vi "AFM_sync_fixed_lightsheet.vi"() -> ()   [LabVIEW 2017]
uses:
  <vilib>/DAQmx/write.llb/DAQmx Write (Analog DBL 1Chan 1Samp).vi
  <vilib>/DAQmx/write.llb/DAQmx Write (Analog 2D DBL NChan NSamp).vi
  <vilib>/DAQmx/create/channels.llb/DAQmx Create Channel (AO-Voltage-Basic).vi
  <vilib>/DAQmx/miscellaneous.llb/DAQmx Fill In Error Info.vi
  <vilib>/DAQmx/create/channels.llb/DAQmx Create Channel (CO-Pulse Generation-Frequency).vi
  <vilib>/DAQmx/configure/timing.llb/DAQmx Timing (Implicit).vi
  <vilib>/DAQmx/configure/trigger.llb/DAQmx Start Trigger (Digital Edge).vi
  <vilib>/DAQmx/configure/timing.llb/DAQmx Timing (Sample Clock).vi
  <resource>/objmgr/daqmx.rc
panel:
  in  "Unit Time":dbl=100.0 caption="ms" format="%#_13g"
  in  "ETL3 (V)  (4.76V allows light passing through unaltered.)":dbl(slide)=4.76 caption="ETL3 (dpt)" min=-12.029999732971191 max=16.450000762939453 step=0.009999999776482582 scale=0.0..10.0
  out "Focal Distance (um)":dbl
  out "Diopter":dbl
  in  "Blanking (0-10V)":dbl=10.0 min=0.0 max=10.0 step=0.1 format="%#_13g"
  in  "561 (0-10V)":dbl=2.0 min=0.0 max=10.0 step=0.1 format="%#_13g"
  in  "488 (0-10V)":dbl=2.0 min=0.0 max=10.0 step=0.1 format="%#_13g"
  out "Matched AFM frequency":dbl caption="frames/s"
  in  "OFF Time Unit":dbl=1.0 caption="(400 ms)" format="%#_13g"
  in  "ON Time Unit":dbl=3.0 caption="(600 ms)" format="%#_13g"
  # "(There is a hidden -1ms in Unit Time)"
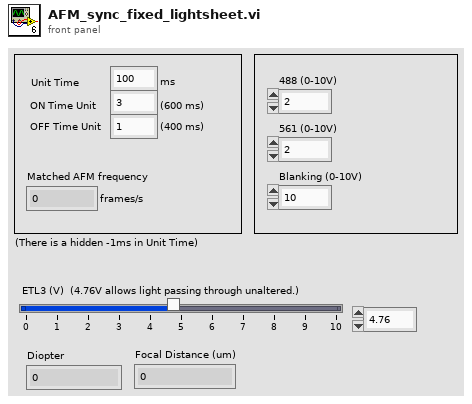
[diagram p1: front panel]
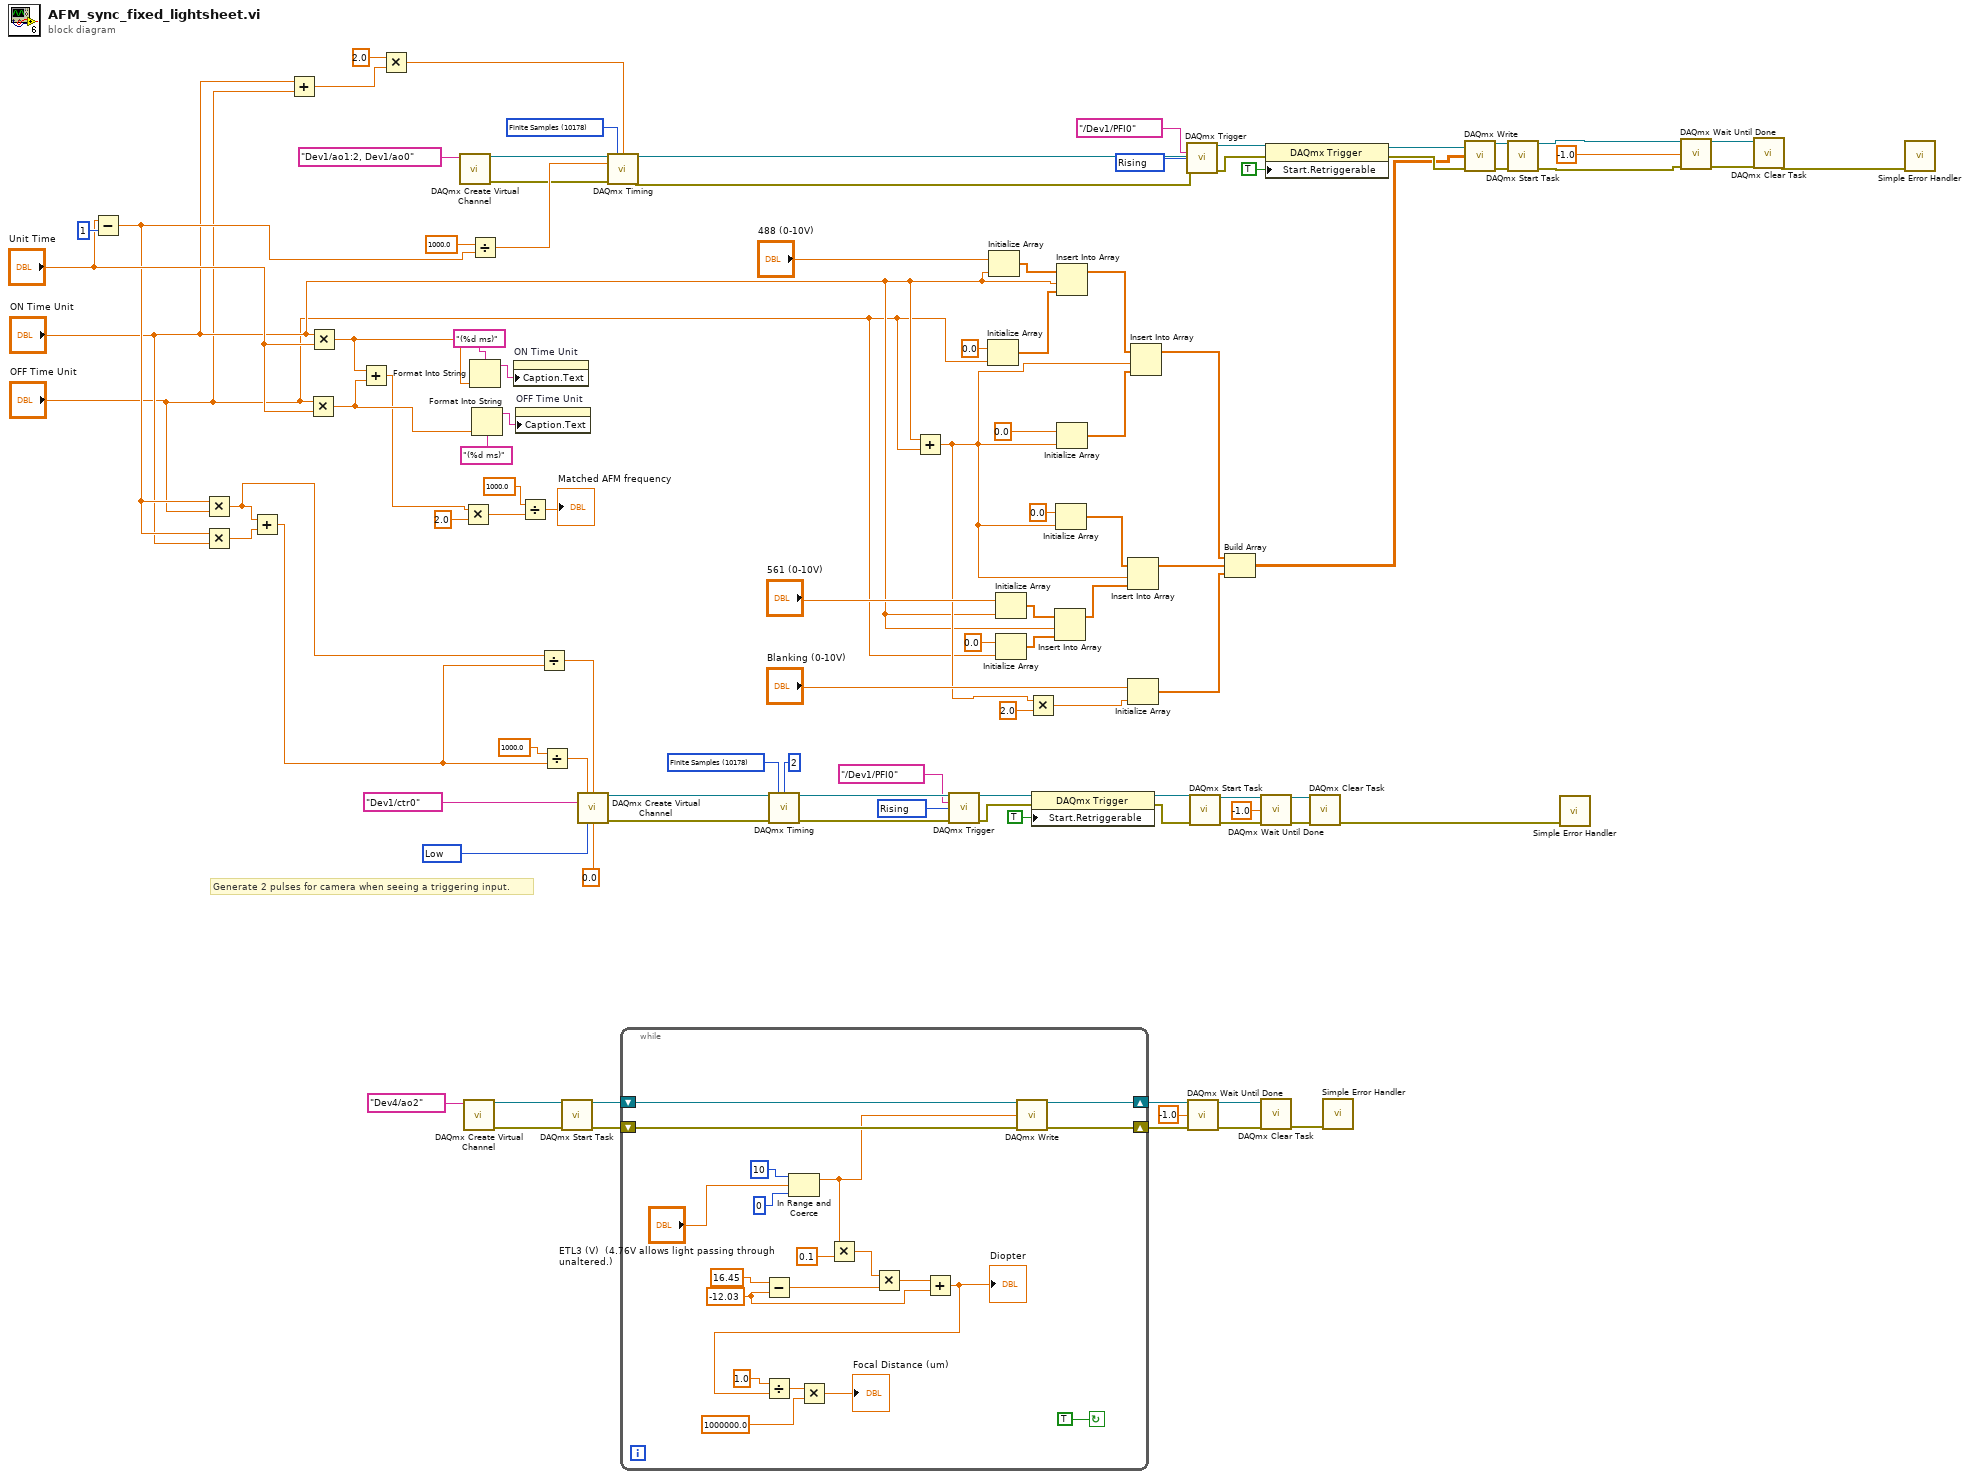
[diagram p0: block diagram]
diagram:
  w69 = 10280 items=["Rising"=10280, "Falling"=10171] ("edge")
  w81 = 10178 items=["Finite Samples"=10178, "Continuous Samples"=10123, "Hardware Timed Single Point"=12522] ("sample mode")
  w91 = 10280 items=["Rising"=10280, "Falling"=10171] ("edge")
  w93 = 10214 items=["High"=10192, "Low"=10214] ("idle state")
  w96 = 10178 items=["Finite Samples"=10178, "Continuous Samples"=10123, "Hardware Timed Single Point"=12522] ("sample mode")
  # "Generate 2 pulses for camera when seeing a triggering input."
  n1 = Subtract(x="Unit Time", y=1 ("samples per channel")) -> (x-y=w6:dbl)
  n2 = Multiply(x=w6, y="OFF Time Unit") -> (x*y=w2:dbl)
  n3 = Multiply(x=w6, y="ON Time Unit") -> (x*y=w7:dbl)
  n4 = Add(x=w2, y=w7) -> (x+y=w3:dbl)
  n5 = Add(x="ON Time Unit", y="OFF Time Unit") -> (x+y=w17:dbl)
  n6 = Multiply(x="OFF Time Unit", y="Unit Time") -> (x*y=w10:dbl)
  n7 = Multiply(x="ON Time Unit", y="Unit Time") -> (x*y=w20:dbl)
  n8 = Add(x=w20, y=w10) -> (x+y=w8:dbl)
  n9 = Multiply(x=2.0, y=w17) -> (x*y=w16:dbl)
  n10 = call-poly <vilib>:"DAQmx Create Virtual Channel.vi"("physical channels"=tag "Dev1/ao1:2, Dev1/ao0") -> ("task out"=w72:refnum<k21>, "error out"=w71:errorcluster)  [unwired: 13 in]
  n11 = Multiply(x=w8, y=2.0) -> (x*y=w42:dbl)
  n12 = call-poly <vilib>:"DAQmx Create Virtual Channel.vi"("physical channels"=tag "Dev4/ao2") -> ("task out"=w31:refnum<k21>, "error out"=w30:errorcluster)  [unwired: 13 in]
  n13 = Divide(x=1000.0, y=w6) -> (x/y=w82:dbl)
  n14 = Format Into String(format string="(%d ms)", w20) -> (resulting string=w27:string)  [unwired: 2 in, 1 out]
  n15 = Format Into String(format string="(%d ms)", w10) -> (resulting string=w26:string)  [unwired: 2 in, 1 out]
  n16 = property on="ON Time Unit" class="DigNum (strict)"("Caption.Text"=w27) -> ()  [unwired: 2 in, 2 out]
  n17 = property on="OFF Time Unit" class="DigNum (strict)"("Caption.Text"=w26) -> ()  [unwired: 2 in, 2 out]
  n18 = Divide(x=1000.0, y=w42) -> (x/y=→"Matched AFM frequency":dbl)
  n19 = Divide(x=w2, y=w3) -> (x/y=w19:dbl)
  n20 = Divide(x=1000.0, y=w3) -> (x/y=w21:dbl)
  n21 = call <vilib>:"DAQmx Start Task.vi"("task/channels in"=w31, "error in"=w30) -> ("task out"=w33:refnum<k21>, "error out"=w32:errorcluster)  [unwired: 12 in]
  n22 = call-poly <vilib>:"DAQmx Create Virtual Channel.vi"("frequency"=w21, "duty cycle"=w19, "counter"=tag "Dev1/ctr0", "idle state"=w93, "initial delay"=0.0) -> ("task out"=w61:refnum<k21>, "error out"=w60:errorcluster)  [unwired: 9 in]
  n23 = call-poly <vilib>:"DAQmx Timing.vi"("task/channels in"=w72, "sample mode"=w81, "samples per channel"=w16, "rate"=w82, "error in"=w71) -> ("task out"=w68:refnum<k21>, "error out"=w67:errorcluster)  [unwired: 9 in]
  n24 = while {
    shift-right: [w121] -> w28
    shift-left: w33 -> [w123]
    shift-right: [w120] -> w29
    shift-left: w32 -> [w122]
    stop <- TRUE continue-if-true
    w105 = -12.03 ("x")
    n25 = Subtract(x=16.45 ("y"), y=w105) -> (x-y=w107:dbl)
    n26 = In Range and Coerce(upper limit=10, x="ETL3 (V)  (4.76V allows light passing through unaltered.)", lower limit=0) -> (coerced(x)=w110:dbl)  [unwired: 1 out]
    n27 = Multiply(x=w110, y=0.1) -> (x*y=w108:dbl)
    n28 = Multiply(x=w108, y=w107) -> (x*y=w106:dbl)
    n29 = Add(x=w106, y=w105) -> (x+y=w104:dbl)
    "Diopter" <- w104
    n30 = Divide(x=1.0, y=w104) -> (x/y=w117:dbl)
    n31 = Multiply(x=w117, y=1000000.0) -> (x*y=→"Focal Distance (um)":dbl)
    n32 = call-poly <vilib>:"DAQmx Write.vi"("task/channels in"=w123, "data"=w110, "error in"=w122) -> ("task out"=w121:refnum<k21>, "error out"=w120:errorcluster)  [unwired: 10 in, 1 out]
  }
  n33 = call-poly <vilib>:"DAQmx Timing.vi"("task/channels in"=w61, "sample mode"=w96, "samples per channel"=2, "error in"=w60) -> ("task out"=w102:refnum<k21>, "error out"=w103:errorcluster)  [unwired: 10 in]
  n34 = Add(x="ON Time Unit", y="OFF Time Unit") -> (x+y=w12:dbl)
  n35 = call-poly <vilib>:"DAQmx Trigger.vi"("task/channels in"=w102, "source"=tag "/Dev1/PFI0", "edge"=w91, "error in"=w103) -> ("task out"=w89:refnum<k21>, "error out"=w87:errorcluster)  [unwired: 10 in]
  n36 = Initialize Array(0.0 ("element"), "OFF Time Unit") -> (w57:dbl[])
  n37 = Initialize Array("488 (0-10V)", "ON Time Unit") -> (w58:dbl[])
  n38 = Initialize Array("561 (0-10V)", "ON Time Unit") -> (w53:dbl[])
  n39 = Initialize Array(0.0 ("element"), "OFF Time Unit") -> (w52:dbl[])
  n40 = Multiply(x=w12, y=2.0) -> (x*y=w41:dbl)
  n41 = property class="DAQmx Trigger"(reference=w89, error in=w87, "Start.Retriggerable"=TRUE) -> (reference out=w88:refnum<k21>, error out=w86:errorcluster)
  n42 = Insert Into Array(array=w53, index="ON Time Unit", new element=w52) -> (w48:dbl[])
  n43 = Initialize Array(0.0 ("element"), w12) -> (w49:dbl[])
  n44 = Insert Into Array(array=w58, index="ON Time Unit", new element=w57) -> (w51:dbl[])
  n45 = Initialize Array(0.0 ("element"), w12) -> (w50:dbl[])
  n46 = Insert Into Array(array=w49, index=w12, new element=w48) -> (w46:dbl[])
  n47 = Initialize Array("Blanking (0-10V)", w41) -> (w45:dbl[])
  n48 = Insert Into Array(array=w51, index=w12, new element=w50) -> (w47:dbl[])
  n49 = call-poly <vilib>:"DAQmx Trigger.vi"("task/channels in"=w68, "source"=tag "/Dev1/PFI0", "edge"=w69, "error in"=w67) -> ("task out"=w65:refnum<k21>, "error out"=w62:errorcluster)  [unwired: 10 in]
  n50 = call <vilib>:"DAQmx Wait Until Done.vi"("task/channels in"=w28, "timeout (sec)"=-1.0, "error in"=w29) -> ("task out"=w37:refnum<k21>, "error out"=w36:errorcluster)  [unwired: 11 in]
  n51 = call <vilib>:"DAQmx Start Task.vi"("task/channels in"=w88, "error in"=w86) -> ("task out"=w97:refnum<k21>, "error out"=w98:errorcluster)  [unwired: 12 in]
  n52 = Build Array(w47, w46, w45) -> (w44:dbl[][])
  n53 = call <vilib>:"DAQmx Wait Until Done.vi"("task/channels in"=w97, "timeout (sec)"=-1.0, "error in"=w98) -> ("task out"=w100:refnum<k21>, "error out"=w99:errorcluster)  [unwired: 11 in]
  n54 = call <vilib>:"DAQmx Clear Task.vi"("task in"=w37, "error in"=w36) -> ("error out"=w38:errorcluster)  [unwired: 13 in]
  n55 = property class="DAQmx Trigger"(reference=w65, error in=w62, "Start.Retriggerable"=TRUE) -> (reference out=w64:refnum<k21>, error out=w63:errorcluster)
  n56 = call <vilib>:"DAQmx Clear Task.vi"("task in"=w100, "error in"=w99) -> ("error out"=w39:errorcluster)  [unwired: 13 in]
  n57 = call <vilib>:"Simple Error Handler.vi"("error in (no error)"=w38) -> ()  [unwired: 4 in, 5 out]
  n58 = call-poly <vilib>:"DAQmx Write.vi"("task/channels in"=w64, "data"=w44, "error in"=w63) -> ("task out"=w75:refnum<k21>, "error out"=w74:errorcluster)  [unwired: 10 in, 1 out]
  n59 = call <vilib>:"DAQmx Start Task.vi"("task/channels in"=w75, "error in"=w74) -> ("task out"=w77:refnum<k21>, "error out"=w78:errorcluster)  [unwired: 12 in]
  n60 = call <vilib>:"Simple Error Handler.vi"("error in (no error)"=w39) -> ()  [unwired: 4 in, 5 out]
  n61 = call <vilib>:"DAQmx Wait Until Done.vi"("task/channels in"=w77, "timeout (sec)"=-1.0, "error in"=w78) -> ("task out"=w80:refnum<k21>, "error out"=w79:errorcluster)  [unwired: 11 in]
  n62 = call <vilib>:"DAQmx Clear Task.vi"("task in"=w80, "error in"=w79) -> ("error out"=w84:errorcluster)  [unwired: 13 in]
  n63 = call <vilib>:"Simple Error Handler.vi"("error in (no error)"=w84) -> ()  [unwired: 4 in, 5 out]
